vi "Upper Term.vi"(11 "Terms[]":refnum<vi>[](array[refnum])) -> (3 "Terms[] out":refnum<vi>)   [LabVIEW 2017, in "CSM-Helper.lvclass"]
uses:
  CSM-Helper.lvclass
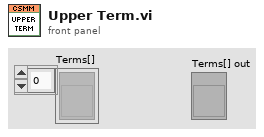
[diagram p1: front panel]
types:
  T1 = typedef "LVPositionTypeDef.ctl" = cluster{"Left":i32, "Top":i32}
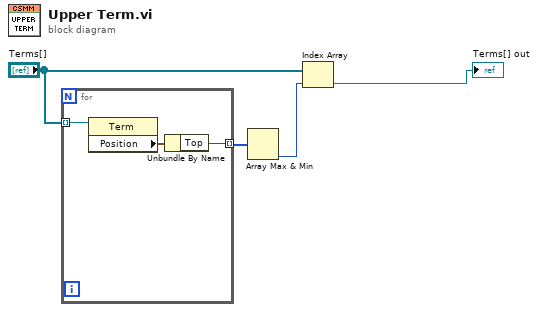
[diagram p0: block diagram]
diagram:
  n1 = for {
    tunnel: "Terms[]" -> [w7] mode=indexing
    tunnel: [w5] -> w4 mode=indexing
    n2 = property class="Term"(reference=w7) -> ("Position"=w6:T1)  [unwired: 1 in, 2 out]
    n3 = Unbundle By Name(w6) -> ("Top"=w5:i32)
  }
  n4 = Array Max & Min(array=w4) -> (min index (indices)=w2:i32)  [unwired: 3 out]
  n5 = Index Array(array="Terms[]", index=w2) -> (element=→"Terms[] out":refnum<vi>)
